vi "Main.vi"() -> ()   [LabVIEW 2026]
doc: "This template is for the Queued Message Handler design pattern.\n\nThe Event Handling Loop generates messages based on user interface actions.\n\nThe Message Handling Loop processes messages generated by the Event Handling Loop, or by other messages. The messages are string values, so new messages can be added easily to the Message Cases case structure in the Message Handling Loop. Each message cluster can also provide an optional value for Message Data, which is a variant that can be converted to whatever message-specific data is required."
uses:
  controls/Controls.ctl
  controls/Display.ctl
  controls/Simulators.ctl
  controls/UI Data.ctl
  controls/System_Status.ctl
  controls/File_Enum.ctl
  <vilib>/Utility/error.llb/Error Cluster From Error Code.vi
  <vilib>/ErrorRing/Error Ring.xnode
  support/Message Queue/Message Queue.lvlib
  support/User Event - Stop/User Event - Stop.lvlib
panel:
  in  "Simulators":T1 {"Milk Level" scale=0.0..100.0; "Bean Level" scale=0.0..100.0; "Water Level" scale=0.0..100.0}
  out "Display":T2 {"Coffee" scale=0.0..80.0; "Chamber" scale=0.0..80.0}
  in  "Controls":T3 {"Type" scale=0.0..2.0}
  in  "Power Button":bool
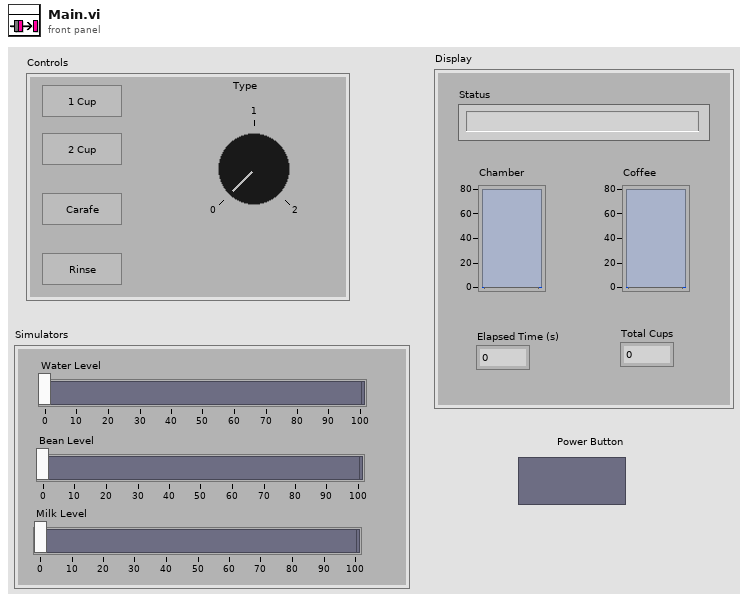
[diagram p1: front panel]
types:
  T1 = typedef "Simulators.ctl" = cluster{"Water Level":dbl, "Bean Level":dbl, "Milk Level":dbl}
  T2 = typedef "Display.ctl" = cluster{"Status":string, "Chamber":dbl, "Coffee":dbl, "Elapsed Time (s)":dbl, "Total Cups":dbl}
  T3 = typedef "Controls.ctl" = cluster{"1 Cup":bool, "2 Cup":bool, "Carafe":bool, "Rinse":bool, "Type":i16}
  T4 = typedef "UI Data.ctl" = cluster{"Simulators":T1, "Controls":T3, "Display":T2, "Power Button":bool, "Simulators Ref":refnum<vi>, "Controls Ref":refnum<vi>, "Display Ref":refnum<vi>, "System Status":T5, "Shutdown?":bool, "Time Remaining":dbl, "Time Target":dbl}
  T5 = typedef "System_Status.ctl" = enum16{"Resetting", "Heating Up", "Rinsing", "Ready for Brewing", "Grinding", "Brewing", "Dispensing", "Shutting Down"}
  T6 = typedef "Message Queue.lvlib/All Message Queues.ctl" = cluster{"UI":refnum<queue>}
  T7 = typedef "File_Enum.ctl" = enum16{"Read", "Write"}
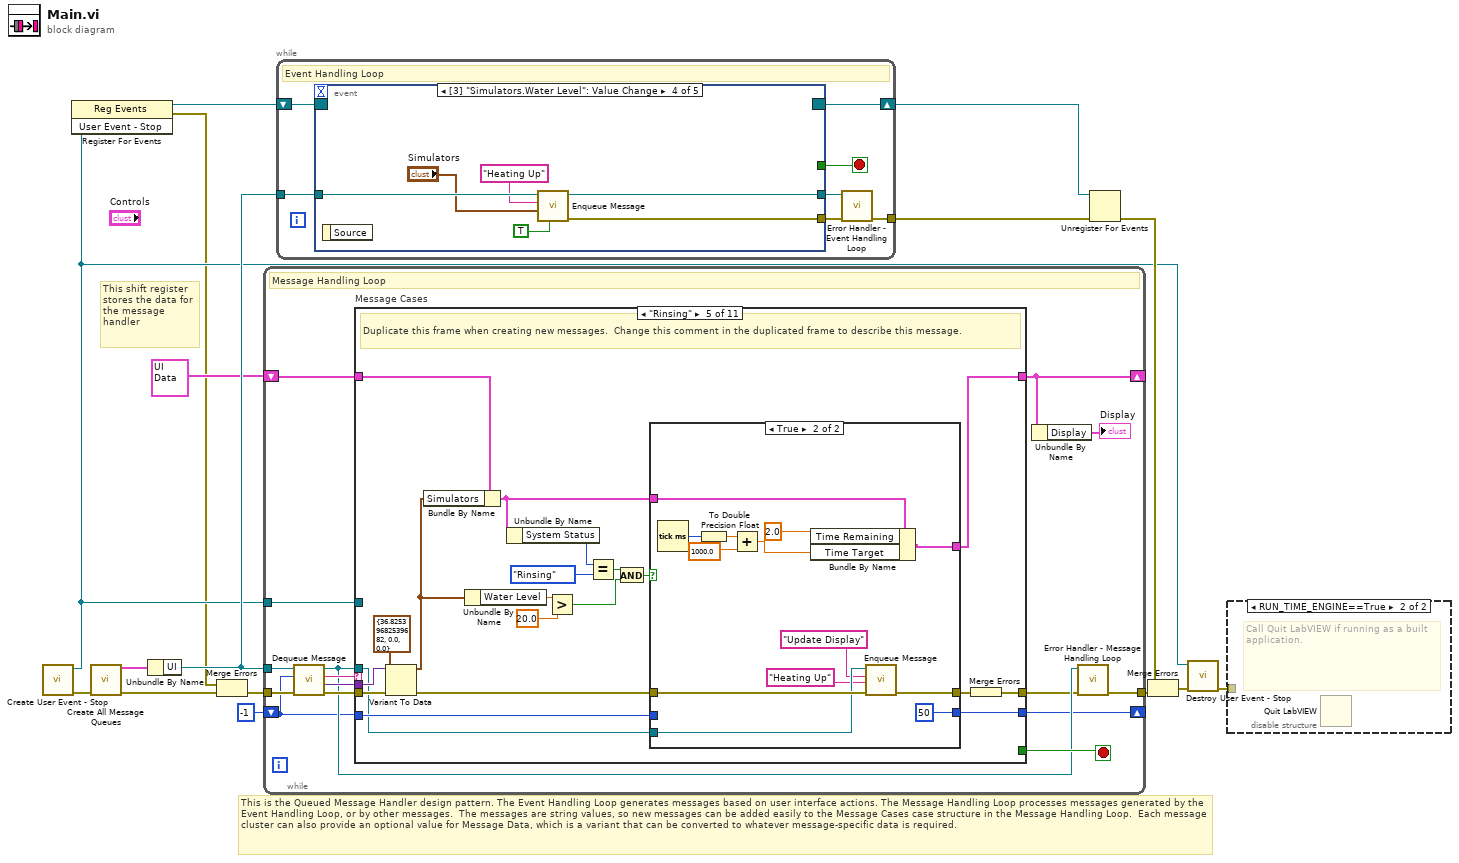
[diagram p0: block diagram]
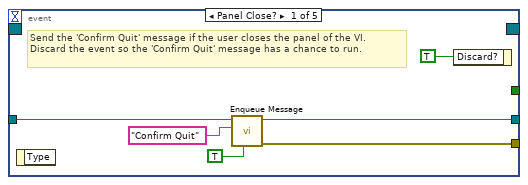
[diagram p3: hidden frame]
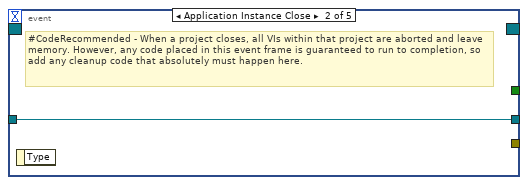
[diagram p4: hidden frame]
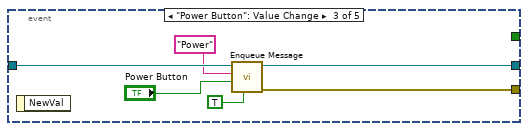
[diagram p5: hidden frame]
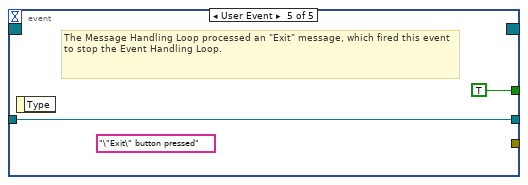
[diagram p6: hidden frame]
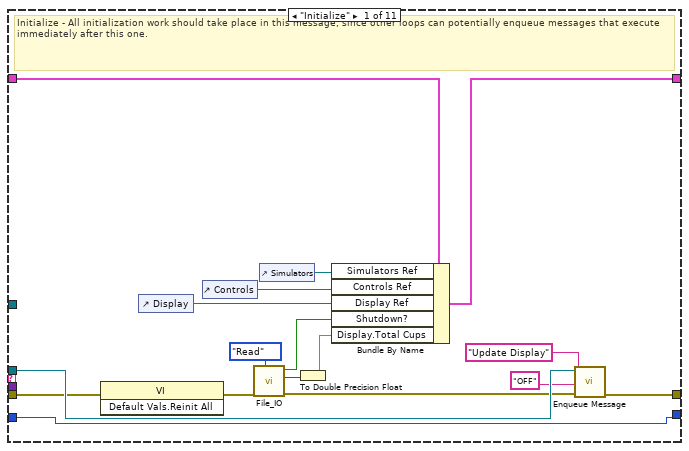
[diagram p7: hidden frame]
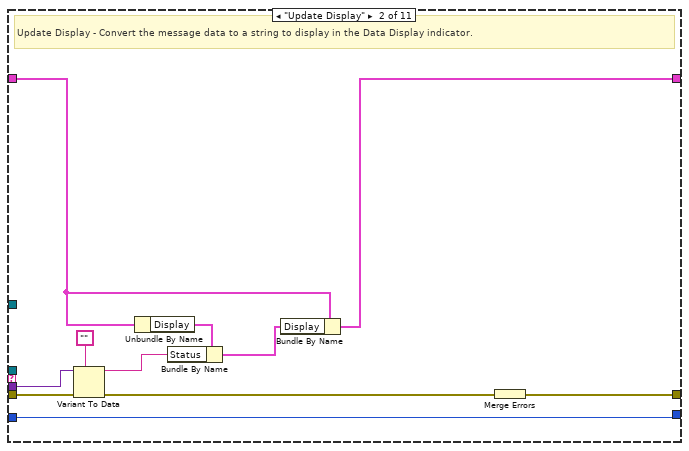
[diagram p8: hidden frame]
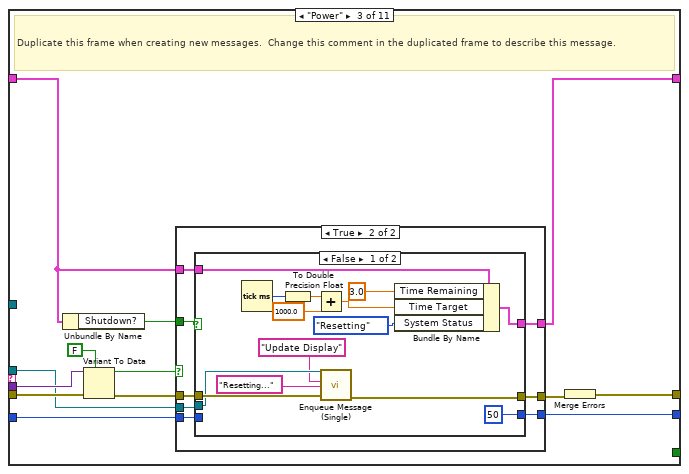
[diagram p9: hidden frame]
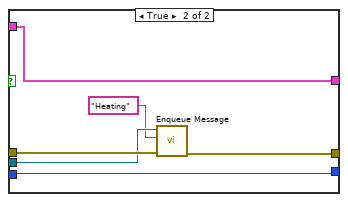
[diagram p11: hidden frame]
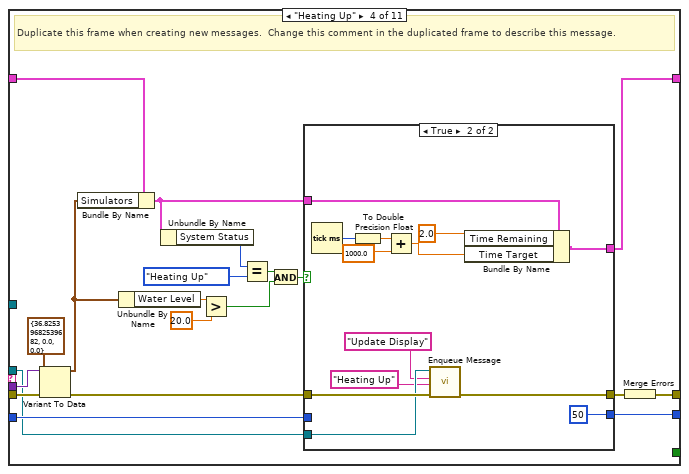
[diagram p12: hidden frame]
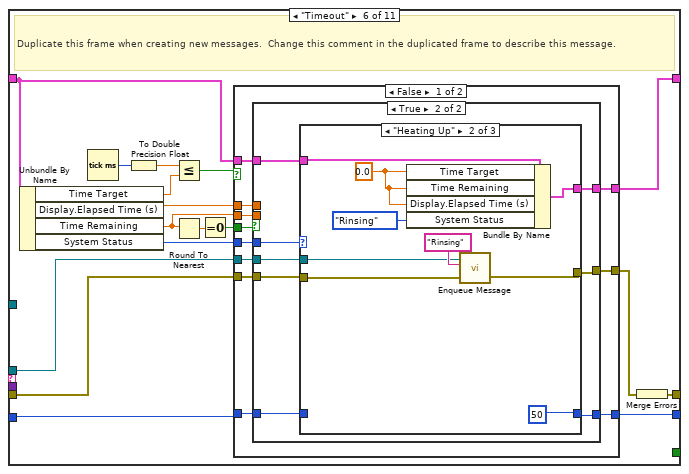
[diagram p15: hidden frame]
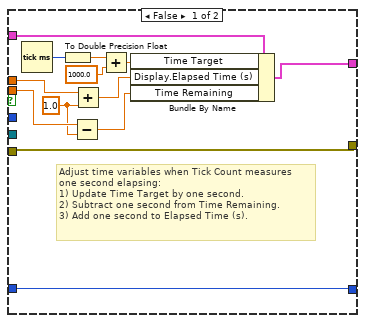
[diagram p16: hidden frame]
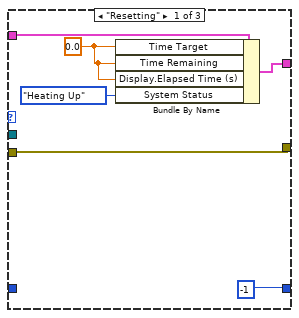
[diagram p17: hidden frame]
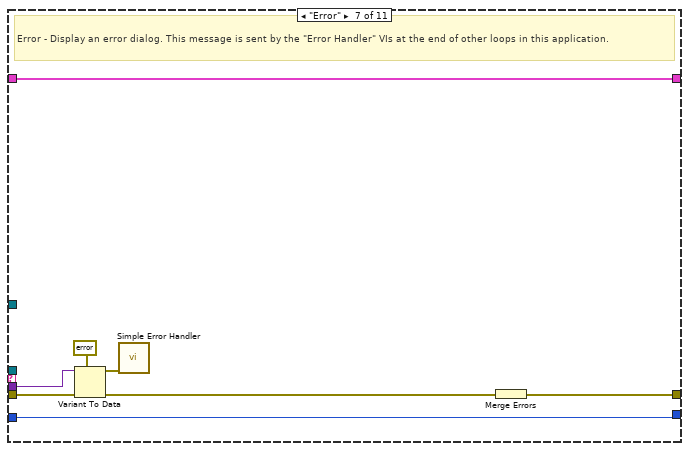
[diagram p20: hidden frame]
diagram:
  # "This is the Queued Message Handler design pattern. The Event Handling Loop generates messages based on user interface actions. The Message Handling Loop processes messages generated by the Event Handling Loop, or by other messages.  The messages are string values, so new messages can be added easily to the Message Cases case structure in the Message Handling Loop.  Each message cluster can also provide an optional value for Message Data, which is a variant that can be converted to whatever message-specific data is required."
  # "This shift register stores the data for the message handler"
  n1 = call "Create User Event - Stop.vi"() -> ("error out"=w12:errorcluster, "User Event - Stop"=w4:refnum<user-event>)  [unwired: 10 in]
  n2 = register-events(w4) -> (reference out=w5:refnum<event-registration>, error out=w2:errorcluster)  [unwired: 2 in]
  n3 = call "Create All Message Queues.vi"("error in (no error)"=w12) -> ("error out"=w16:errorcluster, "Message Queues out"=w15:T6)  [unwired: 9 in]
  n4 = Unbundle By Name(w15) -> ("UI"=w13:refnum<queue>)
  n5 = Merge Errors(w2, w16) -> (w3:errorcluster)
  n6 = while {
    tunnel: w13 -> [w24]
    shift-right: [w20] -> _
    shift-left: T4 {"Simulators"={"Water Level"=0.0, "Bean Level"=0.0, "Milk Level"=0.0}, "Controls"={"1 Cup"=FALSE, "2 Cup"=FALSE, "Carafe"=FALSE, "Rinse"=FALSE, "Type"=0}, "Display"={"Status"="", "Chamber"=0.0, "Coffee"=0.0, "Elapsed Time (s)"=0.0, "Total Cups"=0.0}, "Power Button"=FALSE, "Simulators Ref"=refnum, "Controls Ref"=refnum, "Display Ref"=refnum, "System Status"=enum."Resetting", "Shutdown?"=FALSE, "Time Remaining"=0.0, "Time Target"=0.0} ("Data Cluster") -> [w31]
    tunnel: w4 -> [w29]
    tunnel: w3 -> [w28]
    tunnel: [w22] -> w14
    shift-right: [w18] -> _
    shift-left: -1 -> [w17]
    stop <- w30 stop-if-true
    # "Message Handling Loop"
    n7 = call "Dequeue Message.vi"("error in (no error)"=w28, "timeout in ms (-1)"=w17, "Message Queue"=w24) -> ("error out"=w27:errorcluster, "Message Data"=w25:variant, "Message"=w26:string, "dup Message Queue"=w23:refnum<queue>)  [unwired: 5 in]
    n8 = case "Message Cases" shown="\"Rinsing\"" w26 {
      selector: w26 -> [_ _ _ _ _ _ _ _ _ _ w279]
      tunnel: w23 -> [w44 _ w67 w104 w140 w188 _ w257 _ w277 _]
      tunnel: w27 -> [w42 w58 w71 w117 w153 w187 w253 w261 w265 w270 _]
      tunnel: [w48 w59 w72 w123 w159 w192 w247 w259 w263 w273 w280] -> w21
      tunnel: w31 -> [w47 w52 w62 w112 w148 w182 w252 w260 w264 w276 w281]
      tunnel: [w46 w50 w61 w119 w155 w181 w252 w260 w264 w276 w281] -> w20
      tunnel: [_ _ _ _ _ _ _ _ _ TRUE _] -> w30
      tunnel: w25 -> [_ w57 w70 w114 w150 _ w251 _ _ w267 _]
      tunnel: w29 -> [_ _ _ _ _ _ _ _ _ w272 _]
      tunnel: [w32 w49 w63 w122 w158 w180 w246 w254 w262 w266 w278] -> w18
      tunnel: w17 -> [w32 w49 w60 w120 w156 w179 w246 w254 w262 w266 w278]
      frame "Initialize" {
        # "Initialize - All initialization work should take place in this message, since other loops can potentially enqueue messages that execute immediately after this one."
        n9 = invoke class="VI" method="Default Vals.Reinit All"(error in=w42) -> (error out=w41:errorcluster)  [unwired: 2 in, 2 out]
        n10 = control-ref of="Display"() -> (w37:refnum<vi>)
        n11 = control-ref of="Controls"() -> (w36:refnum<vi>)
        n12 = call "File_IO.vi"("File Enum"=File_Enum."Read", "error in (no error)"=w41) -> ("error out"=w40:errorcluster, "Total Cups Out"=w35:i32, "Shutdown? Out"=w34:bool)  [unwired: 7 in]
        n13 = control-ref of="Simulators"() -> (w38:refnum<vi>)
        n14 = To Double Precision Float(number=w35) -> (double precision float=w33:dbl)
        n15 = Bundle By Name(cluster=w47, "Simulators Ref"=w38, "Controls Ref"=w36, "Display Ref"=w37, "Shutdown?"=w34, "Display.Total Cups"=w33) -> (w46:T4)
        n16 = call-poly "Enqueue Message.vi"("error in (no error)"=w40, "Message Data"="OFF" ("Message"), "Message"="Update Display", "Message Queue"=w44) -> ("error out"=w48:errorcluster)  [unwired: 6 in, 1 out]
      }
      frame "Update Display" {
        # "Update Display - Convert the message data to a string to display in the Data Display indicator."
        n17 = Variant To Data(error in=w58, type="", Variant=w57) -> (data=w55:string, error out=w53:errorcluster)
        n18 = Unbundle By Name(w52) -> ("Display"=w54:T2)
        n19 = Bundle By Name(cluster=w54, "Status"=w55) -> (w51:T2)
        n20 = Bundle By Name(cluster=w52, "Display"=w51) -> (w50:T4)
        n21 = Merge Errors(w53) -> (w59:errorcluster)
      }
      frame "Power" {
        # "Duplicate this frame when creating new messages.  Change this comment in the duplicated frame to describe this message."
        n22 = Unbundle By Name(w62) -> ("Shutdown?"=w65:bool)
        n23 = Variant To Data(error in=w71, type=FALSE ("Priority Message? (F)"), Variant=w70) -> (data=w64:bool, error out=w68:errorcluster)
        n24 = case shown="True" w64 {
          tunnel: w68 -> [w74 w83]
          tunnel: w67 -> [_ w82]
          tunnel: [w74 w81] -> w66
          tunnel: w65 -> [_ w80]
          tunnel: [w75 w79] -> w63
          tunnel: w62 -> [w73 w78]
          tunnel: [w73 w77] -> w61
          tunnel: w60 -> [w75 w76]
          frame False {
          }
          frame True {
            n25 = case shown="False" w80 {
              tunnel: w83 -> [w97 w103]
              tunnel: w82 -> [w96 w102]
              tunnel: [w93 w100] -> w81
              tunnel: [50 w98] -> w79
              tunnel: w78 -> [w91 w99]
              tunnel: [w89 w99] -> w77
              tunnel: w76 -> [_ w98]
              frame False {
                n26 = Tick Count (ms)() -> (millisecond timer value=w87:u32)
                n27 = To Double Precision Float(number=w87) -> (double precision float=w86:dbl)
                n28 = Add(x=w86, y=1000.0) -> (x+y=w84:dbl)
                n29 = call "Enqueue Message (Single).vi"("error in (no error)"=w97, "Message Data"="Resetting..." ("Message"), "Message"="Update Display", "Message Queue"=w96) -> ("error out"=w93:errorcluster)  [unwired: 6 in, 1 out]
                n30 = Bundle By Name(cluster=w91, "Time Remaining"=3.0, "Time Target"=w84, "System Status"=System_Status."Resetting") -> (w89:T4)
              }
              frame True {
                n31 = call-poly "Enqueue Message.vi"("error in (no error)"=w103, "Message"="Heating", "Message Queue"=w102) -> ("error out"=w100:errorcluster)  [unwired: 7 in, 1 out]
              }
            }
          }
        }
        n32 = Merge Errors(w66) -> (w72:errorcluster)
      }
      frame "Heating Up" {
        # "Duplicate this frame when creating new messages.  Change this comment in the duplicated frame to describe this message."
        n33 = Variant To Data(error in=w117, type=T1 {"Water Level"=36.82539682539682, "Bean Level"=0.0, "Milk Level"=0.0} ("Simulators 2"), Variant=w114) -> (data=w111:T1, error out=w116:errorcluster)
        n34 = Bundle By Name(cluster=w112, "Simulators"=w111) -> (w108:T4)
        n35 = Unbundle By Name(w111) -> ("Water Level"=w113:dbl)
        n36 = Unbundle By Name(w108) -> ("System Status"=w105:T5)
        n37 = Greater?(x=w113, y=20.0) -> (0:w110:bool)
        n38 = Equal?(x=w105, y=System_Status."Heating Up" ("System Status")) -> (x = y?=w107:bool)
        n39 = And(x=w107, y=w110) -> (x .and. y?=w109:bool)
        n40 = case shown="True" w109 {
          tunnel: [w126 50] -> w122
          tunnel: w108 -> [w125 w133]
          tunnel: w120 -> [w126 _]
          tunnel: [w125 w132] -> w119
          tunnel: w116 -> [w124 w131]
          tunnel: [w124 w130] -> w118
          tunnel: w104 -> [_ w129]
          frame False {
          }
          frame True {
            n41 = Tick Count (ms)() -> (millisecond timer value=w137:u32)
            n42 = To Double Precision Float(number=w137) -> (double precision float=w136:dbl)
            n43 = Add(x=w136, y=1000.0) -> (x+y=w134:dbl)
            n44 = call-poly "Enqueue Message.vi"("error in (no error)"=w131, "Message Data"="Heating Up" ("Message"), "Message"="Update Display", "Message Queue"=w129) -> ("error out"=w130:errorcluster)  [unwired: 6 in, 1 out]
            n45 = Bundle By Name(cluster=w133, "Time Remaining"=2.0, "Time Target"=w134) -> (w132:T4)
          }
        }
        n46 = Merge Errors(w118) -> (w123:errorcluster)
      }
      frame "Rinsing" {
        # "Duplicate this frame when creating new messages.  Change this comment in the duplicated frame to describe this message."
        n47 = Variant To Data(error in=w153, type=T1 {"Water Level"=36.82539682539682, "Bean Level"=0.0, "Milk Level"=0.0} ("Simulators 2"), Variant=w150) -> (data=w147:T1, error out=w152:errorcluster)
        n48 = Bundle By Name(cluster=w148, "Simulators"=w147) -> (w144:T4)
        n49 = Unbundle By Name(w147) -> ("Water Level"=w149:dbl)
        n50 = Unbundle By Name(w144) -> ("System Status"=w141:T5)
        n51 = Greater?(x=w149, y=20.0) -> (0:w146:bool)
        n52 = Equal?(x=w141, y=System_Status."Rinsing" ("System Status")) -> (x = y?=w143:bool)
        n53 = And(x=w143, y=w146) -> (x .and. y?=w145:bool)
        n54 = case shown="True" w145 {
          tunnel: [w162 50] -> w158
          tunnel: w144 -> [w161 w169]
          tunnel: w156 -> [w162 _]
          tunnel: [w161 w168] -> w155
          tunnel: w152 -> [w160 w167]
          tunnel: [w160 w166] -> w154
          tunnel: w140 -> [_ w165]
          frame False {
          }
          frame True {
            n55 = Tick Count (ms)() -> (millisecond timer value=w173:u32)
            n56 = To Double Precision Float(number=w173) -> (double precision float=w172:dbl)
            n57 = Add(x=w172, y=1000.0) -> (x+y=w170:dbl)
            n58 = Bundle By Name(cluster=w169, "Time Remaining"=2.0, "Time Target"=w170) -> (w168:T4)
            n59 = call-poly "Enqueue Message.vi"("error in (no error)"=w167, "Message Data"="Heating Up" ("Message"), "Message"="Update Display", "Message Queue"=w165) -> ("error out"=w166:errorcluster)  [unwired: 6 in, 1 out]
          }
        }
        n60 = Merge Errors(w154) -> (w159:errorcluster)
      }
      frame "Timeout" {
        # "Duplicate this frame when creating new messages.  Change this comment in the duplicated frame to describe this message."
        n61 = Unbundle By Name(w182) -> ("Time Target"=w176:dbl, "Display.Elapsed Time (s)"=w178:dbl, "Time Remaining"=w177:dbl, "System Status"=w191:T5)
        n62 = Tick Count (ms)() -> (millisecond timer value=w185:u32)
        n63 = To Double Precision Float(number=w185) -> (double precision float=w184:dbl)
        n64 = Less Or Equal?(x=w184, y=w176) -> (x <= y?=w183:bool)
        n65 = Round To Nearest(number=w177) -> (nearest integer value=w190:dbl)
        n66 = Equal To 0?(x=w190) -> (x = 0?=w189:bool)
        n67 = case shown="False" w183 {
          tunnel: w191 -> [w203 _]
          tunnel: w189 -> [w202 _]
          tunnel: w188 -> [w201 _]
          tunnel: w187 -> [w200 w245]
          tunnel: [w199 w245] -> w186
          tunnel: w182 -> [w198 w244]
          tunnel: [w197 w244] -> w181
          tunnel: w178 -> [w194 _]
          tunnel: [w196 w243] -> w180
          tunnel: w179 -> [w195 w243]
          tunnel: w177 -> [w193 _]
          frame False {
            n68 = case shown="True" w202 {
              tunnel: w203 -> [_ w224]
              tunnel: w201 -> [_ w223]
              tunnel: w200 -> [w214 w222]
              tunnel: [w214 w221] -> w199
              tunnel: [w211 w219] -> w197
              tunnel: w198 -> [w213 w220]
              tunnel: [w210 w218] -> w196
              tunnel: w195 -> [w210 w217]
              tunnel: w194 -> [w208 _]
              tunnel: w193 -> [w207 _]
              frame False {
                w206 = 1.0 ("y")
                # "Adjust time variables when Tick Count measures\none second elapsing:\n1) Update Time Target by one second.\n2) Subtract one second from Time Remaining.\n3) Add one second to Elapsed Time (s)."
                n69 = Tick Count (ms)() -> (millisecond timer value=w216:u32)
                n70 = To Double Precision Float(number=w216) -> (double precision float=w215:dbl)
                n71 = Subtract(x=w207, y=w206) -> (x-y=w205:dbl)
                n72 = Add(x=w208, y=w206) -> (x+y=w204:dbl)
                n73 = Add(x=w215, y=1000.0) -> (x+y=w212:dbl)
                n74 = Bundle By Name(cluster=w213, "Time Target"=w212, "Display.Elapsed Time (s)"=w204, "Time Remaining"=w205) -> (w211:T4)
              }
              frame True {
                n75 = case shown="\"Heating Up\"" w224 {
                  tunnel: w223 -> [_ w231 _]
                  tunnel: w222 -> [w225 w233 w242]
                  tunnel: [w225 w232 w242] -> w221
                  tunnel: w220 -> [w230 w239 w241]
                  tunnel: [w228 w237 w241] -> w219
                  tunnel: [-1 50 w240] -> w218
                  tunnel: w217 -> [_ _ w240]
                  frame "Resetting" {
                    w229 = 0.0 ("Time Target")
                    n76 = Bundle By Name(cluster=w230, "Time Target"=w229, "Time Remaining"=w229, "Display.Elapsed Time (s)"=w229, "System Status"=System_Status."Heating Up") -> (w228:T4)
                  }
                  frame "Heating Up" {
                    w238 = 0.0 ("Time Target")
                    n77 = Bundle By Name(cluster=w239, "Time Target"=w238, "Time Remaining"=w238, "Display.Elapsed Time (s)"=w238, "System Status"=System_Status."Rinsing") -> (w237:T4)
                    n78 = call-poly "Enqueue Message.vi"("error in (no error)"=w233, "Message"="Rinsing", "Message Queue"=w231) -> ("error out"=w232:errorcluster)  [unwired: 7 in, 1 out]
                  }
                  frame Default {
                  }
                }
              }
            }
          }
          frame True {
            # "Pass values thrrough and continue counting."
          }
        }
        n79 = Merge Errors(w186) -> (w192:errorcluster)
      }
      frame "Error" {
        # "Error - Display an error dialog. This message is sent by the \"Error Handler\" VIs at the end of other loops in this application."
        n80 = Variant To Data(error in=w253, type=errorcluster {"status"=FALSE, "code"=0, "source"=""} ("error constant"), Variant=w251) -> (data=w249:errorcluster, error out=w248:errorcluster)
        n81 = call <vilib>:"Simple Error Handler.vi"("error in (no error)"=w249) -> ()  [unwired: 4 in, 5 out]
        n82 = Merge Errors(w248) -> (w247:errorcluster)
      }
      frame "Confirm Quit" {
        # "Confirm Quit - Message that can confirm whether or not the user wants to exit the application."
        n83 = call-poly "Enqueue Message.vi"("Priority Message? (F)"=TRUE, "error in (no error)"=w261, "Message"="Exit", "Message Queue"=w257) -> ("error out"=w258:errorcluster)  [unwired: 6 in, 1 out]
        n84 = Merge Errors(w258) -> (w259:errorcluster)
      }
      frame "---Copy This Frame---" {
        # "Duplicate this frame when creating new messages.  Change this comment in the duplicated frame to describe this message."
        n85 = Merge Errors(w265) -> (w263:errorcluster)
      }
      frame "Exit" {
        # "Stop the VI"
        # "Release the message queue reference"
        # "Exit - Exit the application."
        n86 = Variant To Data(type=errorcluster {"status"=FALSE, "code"=0, "source"=""} ("error constant"), Variant=w267) -> (data=w268:errorcluster)  [unwired: 1 in, 1 out]
        n87 = call <vilib>:"Simple Error Handler.vi"("error in (no error)"=w268) -> ()  [unwired: 4 in, 5 out]
        n88 = call "Fire User Event - Stop.vi"("User Event - Stop"=w272) -> ("error out"=w271:errorcluster)  [unwired: 10 in]
        n89 = Release Queue(queue=w277, error in (no error)=w270) -> (error out=w274:errorcluster)  [unwired: 1 in, 2 out]
        n90 = Merge Errors(w271, w274) -> (w273:errorcluster)
      }
      frame Default {
        # "'Default' case only runs if there is a message that isn't defined in any of the other cases.  Output a programming error."
        n91 = xnode "Error Ring"("parameter 0"=w279) -> ("error out"=w280:errorcluster)
      }
    }
    n92 = Unbundle By Name(w20) -> ("Display"=→"Display":T2)
    n93 = call "Error Handler - Message Handling Loop.vi"("error in (no error)"=w21, "Message Queue"=w23) -> ("dup error in"=w22:errorcluster)  [unwired: 8 in, 1 out]
  }
  n94 = while {
    tunnel: w13 -> [w295]
    shift-right: [w293] -> w9
    shift-left: w5 -> [w294]
    tunnel: [w289] -> w6
    stop <- w291 stop-if-true
    # "Event Handling Loop"
    n95 = event shown="[3] \"Simulators.Water Level\": Value Change" {
      selector: w294 -> [_ _ _ _ _]
      dyn-events: [_ _ _ _ _] -> w293
      timeout: _ -> [_ _ _ _ _]
      tunnel: [_ _ _ _ TRUE ("Discard?")] -> w291
      tunnel: w295 -> [w300 w302 w308 w314 w316]
      tunnel: [w299 _ w307 w313 _] -> w292
      tunnel: [w298 w302 w306 w312 w316] -> w290
      event Panel Close? {
        # "Send the 'Confirm Quit' message if the user closes the panel of the VI. Discard the event so the 'Confirm Quit' message has a chance to run."
        n96 = event-data() -> ()  [unwired: 1 in, 1 out]
        n97 = call-poly "Enqueue Message.vi"("Priority Message? (F)"=TRUE, "Message"="Confirm Quit", "Message Queue"=w300) -> ("error out"=w299:errorcluster, "dup Message Queue"=w298:refnum<queue>)  [unwired: 7 in]
        n98 = event-data("Discard?"=TRUE) -> ()  [unwired: 1 in, 1 out]
      }
      event Application Instance Close {
        # "#CodeRecommended - When a project closes, all VIs within that project are aborted and leave memory. However, any code placed in this event frame is guaranteed to run to completion, so add any cleanup code that absolutely must happen here."
        n99 = event-data() -> ()  [unwired: 1 in, 1 out]
      }
      event "Power Button": Value Change {
        n100 = event-data() -> ()  [unwired: 1 in, 1 out]
        n101 = call-poly "Enqueue Message.vi"("Priority Message? (F)"=TRUE, "Message Data"="Power Button", "Message"="Power", "Message Queue"=w308) -> ("error out"=w307:errorcluster, "dup Message Queue"=w306:refnum<queue>)  [unwired: 6 in]
      }
      event Value Change {
        n102 = event-data() -> ()  [unwired: 1 in, 1 out]
        n103 = call-poly "Enqueue Message.vi"("Priority Message? (F)"=TRUE, "Message Data"="Simulators", "Message"="Heating Up", "Message Queue"=w314) -> ("error out"=w313:errorcluster, "dup Message Queue"=w312:refnum<queue>)  [unwired: 6 in]
      }
      event User Event {
        (unwired) "\"Exit\" button pressed" ("VI Stopped")
        # "The Message Handling Loop processed an \"Exit\" message, which fired this event to stop the Event Handling Loop."
        n104 = event-data() -> ()  [unwired: 1 in, 1 out]
      }
    }
    n105 = call "Error Handler - Event Handling Loop.vi"("error in (no error)"=w292, "Message Queue"=w290) -> ("dup error in"=w289:errorcluster)  [unwired: 8 in, 1 out]
  }
  n106 = Unregister For Events(event registration refnum=w9, error in=w6) -> (error out=w10:errorcluster)
  n107 = Merge Errors(w10, w14) -> (w11:errorcluster)
  n108 = call "Destroy User Event - Stop.vi"("error in (no error)"=w11, "User Event - Stop"=w4) -> ("error out"=w7:errorcluster)  [unwired: 9 in]
  n109 = disable-structure shown="RUN_TIME_ENGINE==True" {
    disable-tunnel: w7 -> [_ _]
    frame condition #0 (active) {
    }
    frame condition #1 {
      # "Call Quit LabVIEW if running as a built application."
      n110 = Quit LabVIEW() -> ()  [unwired: 1 in]
    }
  }
